vi "Close-open permission controls.vi"(8 "error in (no error)":errorcluster, 9 "Boolean":bool, 11 "Control-Client in":refnum<class "Control-Client.lvclass">) -> (0 "error out":errorcluster, 3 "Control-Client out":refnum<class "Control-Client.lvclass">)   [LabVIEW 2015, in "Control-Client.lvclass"]
uses:
  Control-Client.lvclass
  dependecies/ControlsVIs/Clusters-def/Controls-with-permissions_CLIENT.ctl
  controls/DigitalIndicatorELYSEpulses.ctl
  controls/CellsSD.ctl
  controls/CellBoolean.ctl
  dependecies/XControls/CellsDL/ControlDL.xctl
  controls/Gauge_pump/Gauge_pump.xctl
  controls/WCM.ctl
  Control-Client.lvclass/Control-Client.ctl
  GeneralFunctionality/GeneralFunctionality.lvclass/GeneralFunctionality.ctl
  Config/Config.lvclass
  GeneralFunctionality/GeneralFunctionality.lvclass
panel:
  out "output cluster":T1
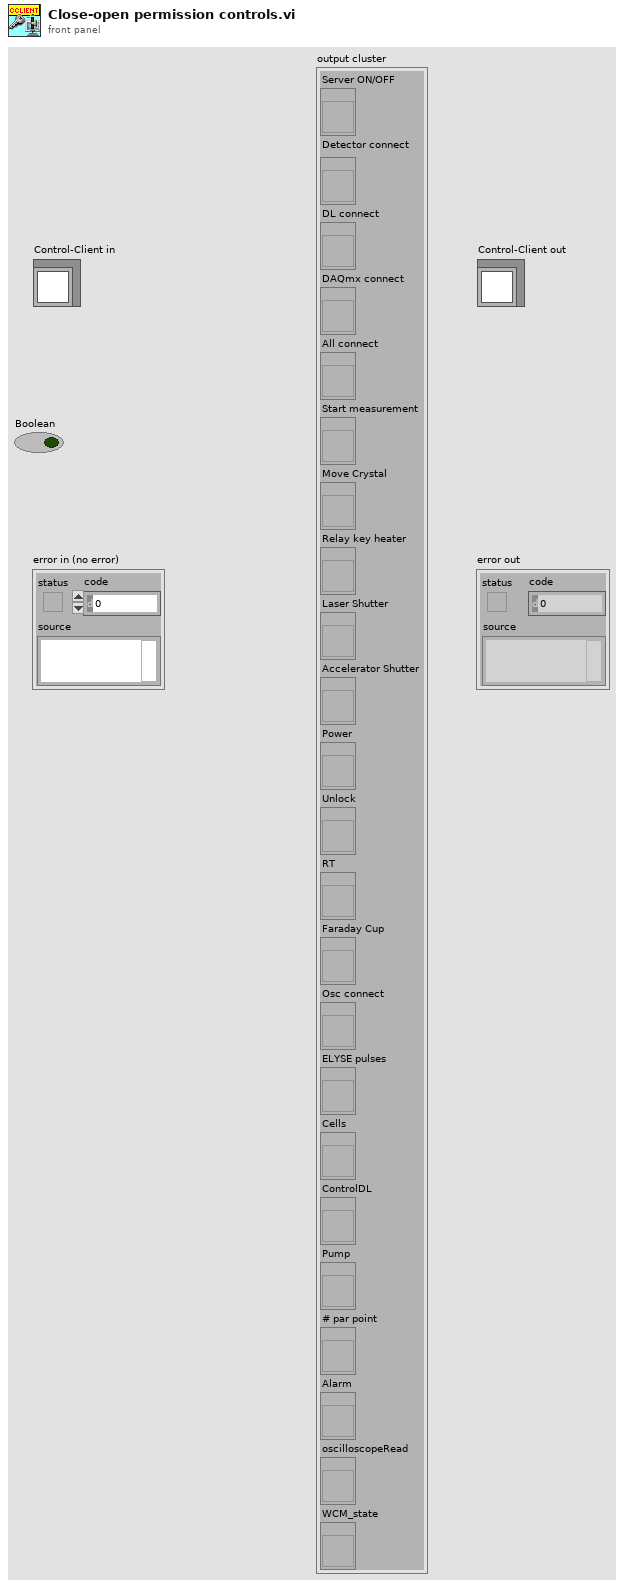
[diagram p1: front panel]
types:
  T1 = typedef "Control-Client.lvclass/Controls-with-permissions_CLIENT.ctl" = cluster{"Server ON/OFF":refnum<vi>, "Detector connect":refnum<vi>, "DL connect":refnum<vi>, "DAQmx connect":refnum<vi>, "All connect":refnum<vi>, "Start measurement":refnum<vi>, "Move Crystal":refnum<vi>, "Relay key heater":refnum<vi>, "Laser Shutter":refnum<vi>, "Accelerator Shutter":refnum<vi>, "Power":refnum<vi>, "Unlock":refnum<vi>, "RT":refnum<vi>, "Faraday Cup":refnum<vi>, "Osc connect":refnum<vi>, "ELYSE pulses":refnum<vi>, "Cells":refnum<vi>, "ControlDL":refnum<vi>, "Pump":refnum<vi>, "# par point":refnum<vi>, "Alarm":refnum<vi>, "oscilloscopeRead":refnum<vi>, "WCM_state":refnum<vi>}
  T2 = enum8{"Enabled", "Disabled", "Disabled and Grayed Out"}
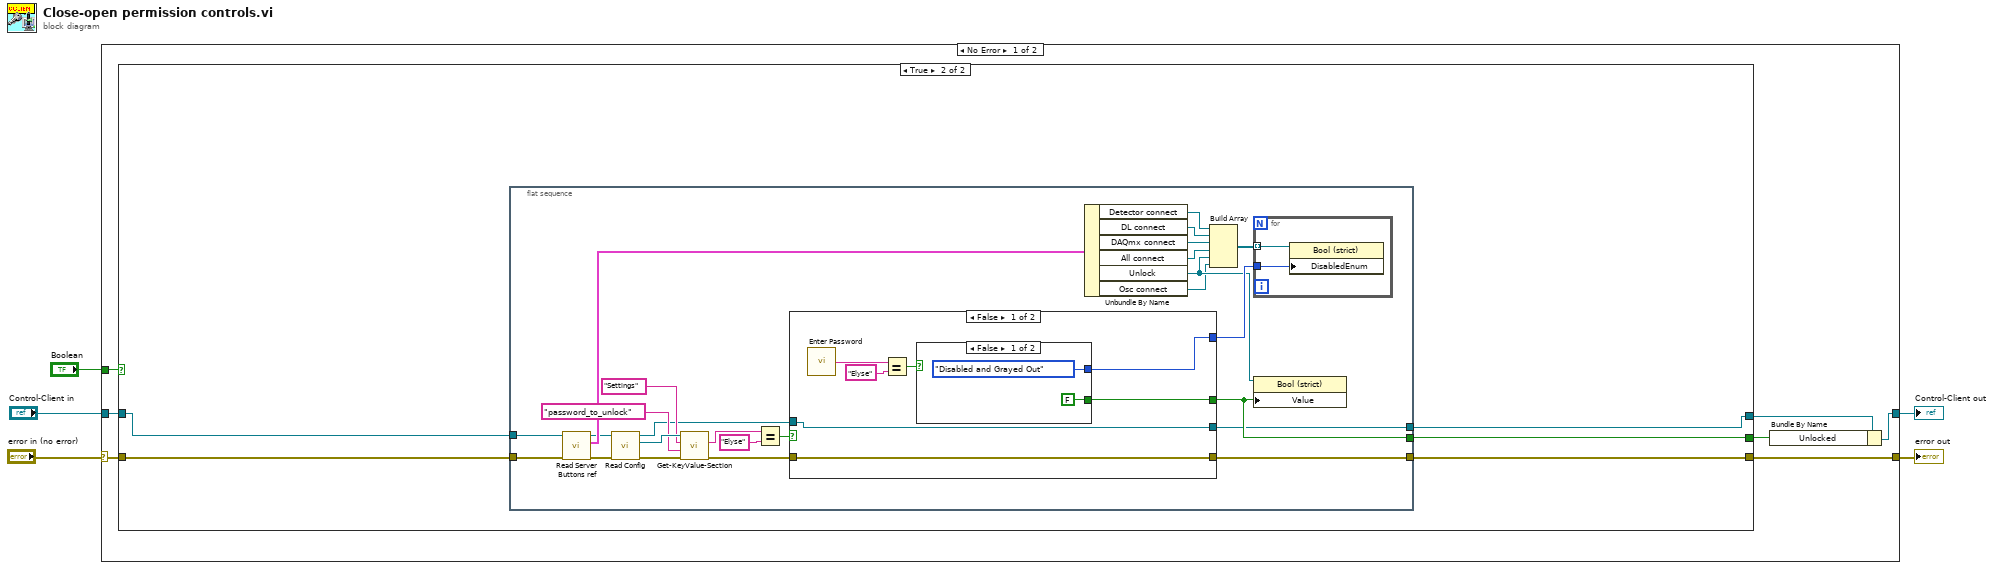
[diagram p0: block diagram]
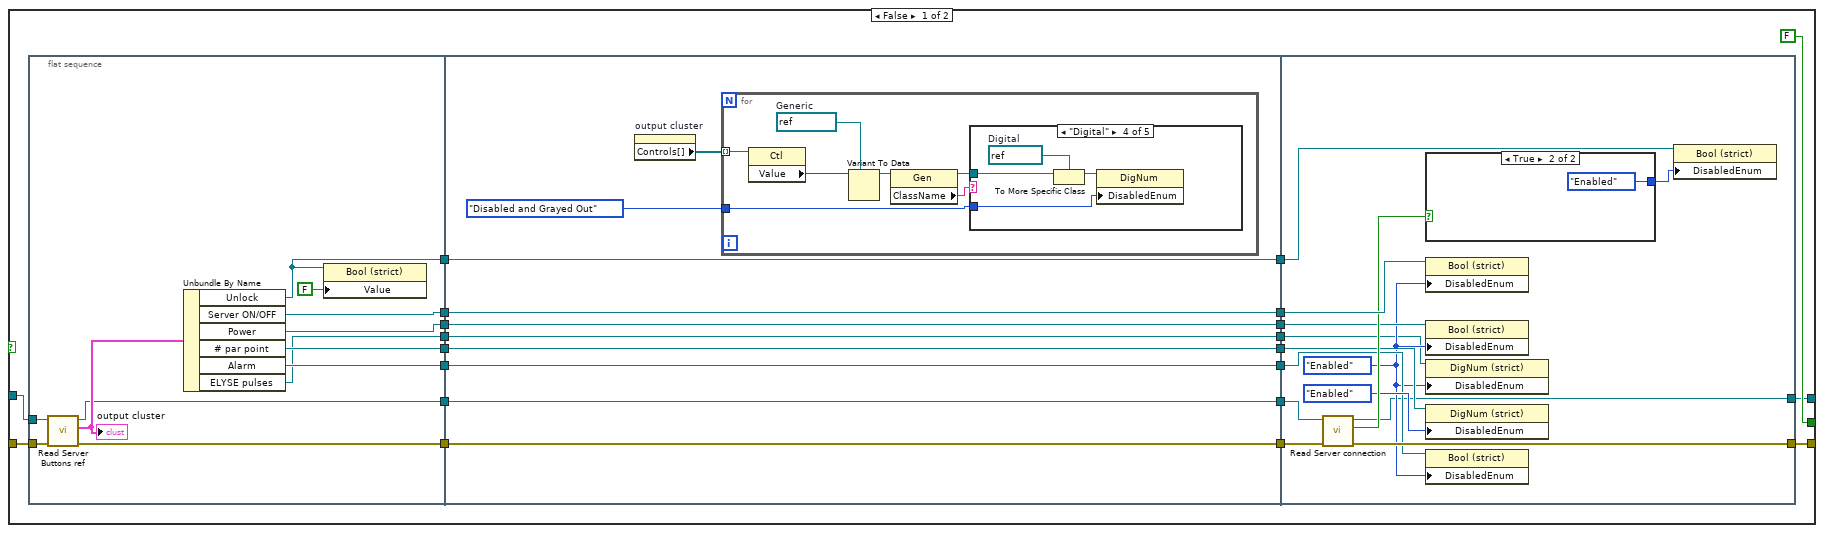
[diagram p2: hidden frame]
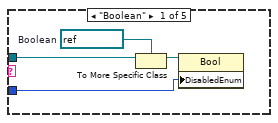
[diagram p3: hidden frame]
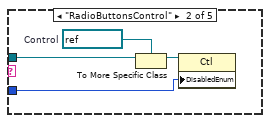
[diagram p4: hidden frame]
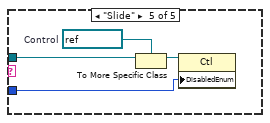
[diagram p6: hidden frame]
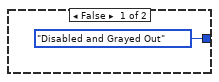
[diagram p7: hidden frame]
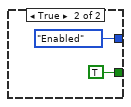
[diagram p8: hidden frame]
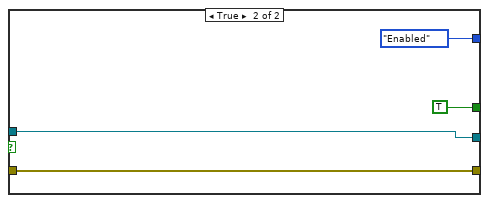
[diagram p9: hidden frame]
diagram:
  n1 = case shown="No Error" "error in (no error)" {
    selector: "error in (no error)" -> [w10 w143]
    tunnel: [w11 w143] -> w4
    tunnel: [w7 w142] -> w2
    tunnel: "Control-Client in" -> [w9 w142]
    tunnel: "Boolean" -> [w12 _]
    frame No Error {
      n2 = case shown="True" w12 {
        tunnel: w9 -> [w33 w96]
        tunnel: w10 -> [w32 w98]
        tunnel: [w31 w99] -> w11
        tunnel: [FALSE w97] -> w8
        tunnel: [w13 w95] -> w6
        frame False {
          n3 = flat-sequence {
            tunnel: w33 -> [w39]
            tunnel: w32 -> [w45]
            tunnel: [w44] -> w30
            tunnel: [w41] -> w27
            tunnel: [w40] -> w25
            tunnel: [w34] -> w23
            tunnel: [w38] -> w22
            tunnel: [w37] -> w18
            tunnel: [w36] -> w17
            tunnel: [w35] -> w14
            tunnel: w30 -> [w55]
            tunnel: [w55] -> w29
            tunnel: [w52] -> w28
            tunnel: w27 -> [w52]
            tunnel: [w51] -> w26
            tunnel: w25 -> [w51]
            tunnel: [w50] -> w24
            tunnel: w23 -> [w50]
            tunnel: w22 -> [w49]
            tunnel: [w49] -> w21
            tunnel: [w48] -> w19
            tunnel: w18 -> [w48]
            tunnel: w17 -> [w47]
            tunnel: [w47] -> w16
            tunnel: [w46] -> w15
            tunnel: w14 -> [w46]
            tunnel: [w88] -> w31
            tunnel: w29 -> [w89]
            tunnel: w28 -> [w92]
            tunnel: w26 -> [w91]
            tunnel: w24 -> [w90]
            tunnel: w21 -> [w85]
            tunnel: w19 -> [w84]
            tunnel: w16 -> [w82]
            tunnel: w15 -> [w80]
            tunnel: [w79] -> w13
            frame #0 {
              n4 = call "Read Server Buttons ref.vi"("error in (no error)"=w45, "Control-Client in"=w39) -> ("error out"=w44:errorcluster, "Server Buttons ref"=w43:T1, "Control-Client out"=w34:refnum<class "Control-Client.lvclass">)  [unwired: 7 in]
              "output cluster" <- w43
              n5 = Unbundle By Name(w43) -> ("Unlock"=w41:refnum<vi>, "Server ON/OFF"=w40:refnum<vi>, "Power"=w38:refnum<vi>, "# par point"=w37:refnum<vi>, "Alarm"=w36:refnum<vi>, "ELYSE pulses"=w35:refnum<vi>)
              n6 = property class="Bool (strict)"(reference=w41, "Value"=FALSE ("Valeur")) -> ()  [unwired: 1 in, 2 out]
            }
            frame #1 {
              n7 = property on="output cluster" class="Clust (strict)"() -> ("Controls[]"=w54:refnum<vi>[])  [unwired: 2 in, 2 out]
              n8 = for {
                tunnel: w54 -> [w62] mode=indexing
                tunnel: T2."Disabled and Grayed Out" ("Disabled") -> [w57]
                w60 = refnum<vi> refnum  # Generic
                n9 = property class="Ctl"(reference=w62) -> ("Value"=w61:variant)  [unwired: 1 in, 2 out]
                n10 = Variant To Data(type=w60, Variant=w61) -> (data=w58:refnum<vi>)  [unwired: 1 in, 1 out]
                n11 = property class="Gen"(reference=w58) -> (reference out=w56:refnum<vi>, "ClassName"=w59:string)  [unwired: 1 in, 1 out]
                n12 = case shown="\"Digital\"" w59 {
                  tunnel: w56 -> [w64 w68 _ w74 w78]
                  tunnel: w57 -> [w63 w67 _ w71 w76]
                  frame "Boolean" {
                    w66 = refnum<vi> refnum  # Boolean
                    n13 = To More Specific Class(target class=w66, reference=w64) -> (specific class reference=w65:refnum<vi>)  [unwired: 1 in, 1 out]
                    n14 = property class="Bool"(reference=w65, "DisabledEnum"=w63) -> ()  [unwired: 1 in, 2 out]
                  }
                  frame "RadioButtonsControl" {
                    w70 = refnum<vi> refnum  # Control
                    n15 = To More Specific Class(target class=w70, reference=w68) -> (specific class reference=w69:refnum<vi>)  [unwired: 1 in, 1 out]
                    n16 = property class="Ctl"(reference=w69, "DisabledEnum"=w67) -> ()  [unwired: 1 in, 2 out]
                  }
                  frame Default {
                  }
                  frame "Digital" {
                    w73 = refnum<vi> refnum  # Digital
                    n17 = To More Specific Class(target class=w73, reference=w74) -> (specific class reference=w72:refnum<vi>)  [unwired: 1 in, 1 out]
                    n18 = property class="DigNum"(reference=w72, "DisabledEnum"=w71) -> ()  [unwired: 1 in, 2 out]
                  }
                  frame "Slide" {
                    w75 = refnum<vi> refnum  # Control
                    n19 = To More Specific Class(target class=w75, reference=w78) -> (specific class reference=w77:refnum<vi>)  [unwired: 1 in, 1 out]
                    n20 = property class="Ctl"(reference=w77, "DisabledEnum"=w76) -> ()  [unwired: 1 in, 2 out]
                  }
                }
              }
            }
            frame #2 {
              w81 = T2."Enabled" ("Désactivé")
              n21 = call "Read Server connection.vi"("error in (no error)"=w89, "Control-Client in"=w90) -> ("error out"=w88:errorcluster, "Server connection"=w87:bool, "Control-Client out"=w79:refnum<class "Control-Client.lvclass">)  [unwired: 7 in]
              n22 = case shown="True" w87 {
                tunnel: [T2."Disabled and Grayed Out" ("Désactivé") T2."Enabled" ("Désactivé")] -> w86
                frame False {
                }
                frame True {
                }
              }
              n23 = property class="Bool (strict)"(reference=w91, "DisabledEnum"=w81) -> ()  [unwired: 1 in, 2 out]
              n24 = property class="Bool (strict)"(reference=w85, "DisabledEnum"=w81) -> ()  [unwired: 1 in, 2 out]
              n25 = property class="DigNum (strict)"(reference=w80, "DisabledEnum"=w81) -> ()  [unwired: 1 in, 2 out]
              n26 = property class="DigNum (strict)"(reference=w84, "DisabledEnum"=T2."Enabled" ("Désactivé")) -> ()  [unwired: 1 in, 2 out]
              n27 = property class="Bool (strict)"(reference=w82, "DisabledEnum"=w81) -> ()  [unwired: 1 in, 2 out]
              n28 = property class="Bool (strict)"(reference=w92, "DisabledEnum"=w86) -> ()  [unwired: 1 in, 2 out]
            }
          }
        }
        frame True {
          n29 = flat-sequence {
            tunnel: [w115] -> w99
            tunnel: w98 -> [w114]
            tunnel: [w112] -> w97
            tunnel: w96 -> [w103]
            tunnel: [w100] -> w95
            frame #0 {
              n30 = call "Read Server Buttons ref.vi"("error in (no error)"=w114, "Control-Client in"=w103) -> ("error out"=w101:errorcluster, "Server Buttons ref"=w111:T1, "Control-Client out"=w102:refnum<class "Control-Client.lvclass">)  [unwired: 7 in]
              n31 = call "Read Config.vi"("error in (no error)"=w101, "GeneralFunctionality en entrée"=w102) -> ("error out"=w123:errorcluster, "Config.lvclass"=w124:refnum<class "Config.lvclass">, "GeneralFunctionality en sortie"=w117:refnum<class "Control-Client.lvclass">)  [unwired: 7 in]
              n32 = call-dynamic "Get-KeyValue-Section.vi"("error in (no error)"=w123, "Key"="password_to_unlock", "Section"="Settings", "Config in"=w124) -> ("error out"=w116:errorcluster, "Value"=w120:string)  [unwired: 5 in, 1 out]
              n33 = Equal?(x=w120, y="Elyse") -> (x = y?=w118:bool)
              n34 = case shown="False" w118 {
                tunnel: [w131 T2."Enabled" ("Disabled")] -> w113
                tunnel: w117 -> [w127 w138]
                tunnel: w116 -> [w129 w140]
                tunnel: [w129 w140] -> w115
                tunnel: [w128 TRUE] -> w112
                tunnel: [w127 w138] -> w100
                frame False {
                  n35 = call "Enter Password.vi"() -> ("Password 2"=w130:string)
                  n36 = Equal?(x=w130, y="Elyse") -> (x = y?=w132:bool)
                  n37 = case shown="False" w132 {
                    tunnel: [T2."Disabled and Grayed Out" ("Disabled") T2."Enabled" ("Disabled")] -> w131
                    tunnel: [FALSE TRUE] -> w128
                    frame False {
                    }
                    frame True {
                    }
                  }
                }
                frame True {
                }
              }
              n38 = Unbundle By Name(w111) -> ("Detector connect"=w109:refnum<vi>, "DL connect"=w108:refnum<vi>, "DAQmx connect"=w107:refnum<vi>, "All connect"=w106:refnum<vi>, "Unlock"=w105:refnum<vi>, "Osc connect"=w104:refnum<vi>)
              n39 = Build Array(w109, w108, w107, w106, w105, w104) -> (w110:refnum<vi>[])
              n40 = for {
                tunnel: w110 -> [w126] mode=indexing
                tunnel: w113 -> [w125]
                n41 = property class="Bool (strict)"(reference=w126, "DisabledEnum"=w125) -> ()  [unwired: 1 in, 2 out]
              }
              n42 = property class="Bool (strict)"(reference=w105, "Value"=w112) -> ()  [unwired: 1 in, 2 out]
            }
          }
        }
      }
      n43 = Bundle By Name(cluster=w6, "Unlocked"=w8) -> (w7:refnum<class "Control-Client.lvclass">)
    }
    frame Error {
    }
  }
  "error out" <- w4
  "Control-Client out" <- w2
